vi "testing_DVR_in_UserEvent.vi"() -> ()   [LabVIEW 2019, in "Service.lvlib"]
uses:
  mmw_service/src_LabVIEW/lib/mmw_Service/Service.lvlib
panel:
  in  "data in":dbl
  out "data value":dbl
  in  "send":bool
  in  "stop":bool
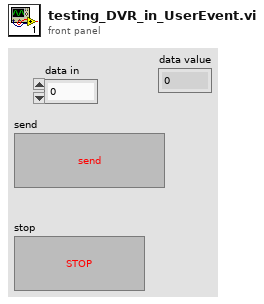
[diagram p1: front panel]
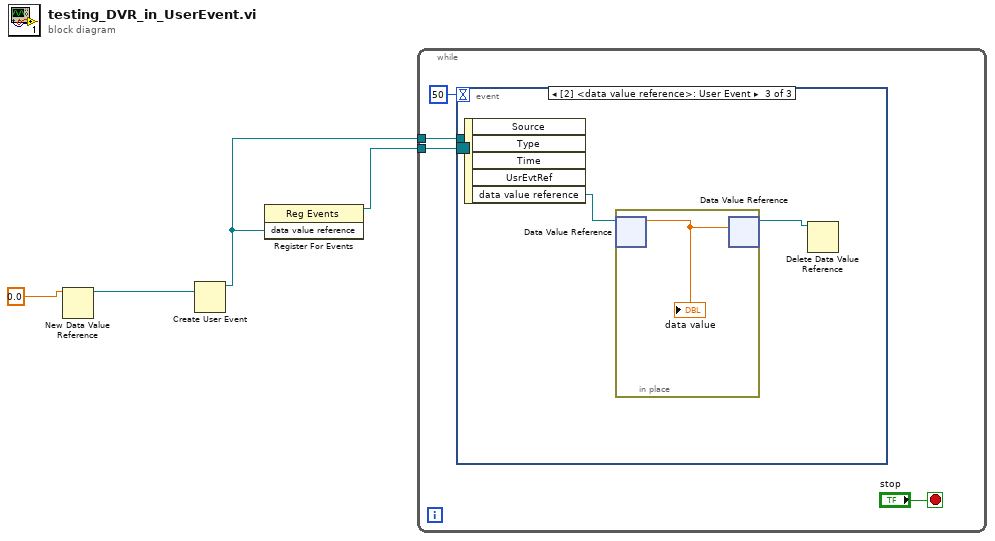
[diagram p0: block diagram]
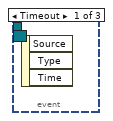
[diagram p2: hidden frame]
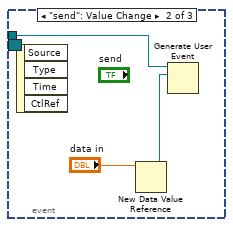
[diagram p3: hidden frame]
diagram:
  n1 = New Data Value Reference(data value=0.0) -> (data value reference=w3:refnum<data-value>)  [unwired: 1 in, 1 out]
  n2 = Create User Event(user event datatype=w3) -> (user event=w1:refnum<user-event>)  [unwired: 1 in, 1 out]
  n3 = register-events(w1) -> (reference out=w2:refnum<event-registration>)  [unwired: 2 in, 1 out]
  n4 = while {
    tunnel: w2 -> [w7]
    tunnel: w1 -> [w6]
    stop <- "stop" stop-if-true
    n5 = event shown="[2] <data value reference>: User Event" {
      selector: w7 -> [_ _ _]
      dyn-events: _ -> [_ _ _]
      timeout: 50 -> [_ _ _]
      tunnel: w6 -> [_ w11 _]
      event Timeout {
        n6 = event-data() -> ()  [unwired: 1 in, 3 out]
      }
      event "send": Value Change {
        n7 = event-data() -> ()  [unwired: 1 in, 4 out]
        n8 = New Data Value Reference(data value="data in") -> (data value reference=w9:refnum<data-value>)  [unwired: 1 in, 1 out]
        n9 = Generate User Event(user event=w11, event data cluster=w9) -> ()  [unwired: 2 in, 2 out]
      }
      event User Event {
        n10 = event-data() -> ("data value reference"=w13:refnum<data-value>)  [unwired: 1 in, 4 out]
        n11 = in-place {
          n12 = in-place-dvr #1(w13) -> (w14:dbl)  [unwired: 1 out]
          "data value" <- w14
          n13 = in-place-dvr #1(w14) -> (w12:refnum<data-value>)  [unwired: 1 out]
        }
        n14 = Delete Data Value Reference(data value reference=w12) -> ()  [unwired: 1 in, 2 out]
      }
    }
  }
